vi "Main Page.vi"(8 "error in (no error)":errorcluster, 11 "Node Ptr":T2 format="%.0x") -> (0 "error out":errorcluster)   [LabVIEW 2024, in "Embedded TDMS Logger System Explorer.lvlib"]
doc: "The UI Page giving the user the ability to modify properties on the file level of the custom device, i.e.:\n- Segmentation options\n- Meta Data to be logged on the file level of the TDMS\n- Naming convention of the file\n- Name of the Custom Device\n- Directory to log files into."
uses:
  Embedded TDMS Logger System Explorer.lvlib
  <vilib>/NI VeriStand/Custom Device API/Custom Device Item Ref.ctl
  Shared/SegmentOptions.ctl
  Shared/File Classes/Meta Data.ctl
  <vilib>/NI VeriStand/Custom Device API/Get Item Property (U16).vi
  <vilib>/NI VeriStand/Custom Device API/Get Item Property (Variant).vi
  <vilib>/NI VeriStand/Custom Device API/Set Item Property (Variant).vi
  <vilib>/NI VeriStand/Custom Device API/Set Item Property (U16).vi
  <vilib>/NI VeriStand/Custom Device API/Set Item Property (String).vi
  <vilib>/NI VeriStand/Custom Device API/Set Item Property (Boolean).vi
  <vilib>/NI VeriStand/Custom Device API/Set Item Property (U64).vi
  <vilib>/NI VeriStand/Custom Device API/Custom Device API.lvlib
panel:
  in  "Tab Control":enum32{"File Settings", "Actions", "Meta Data"}(tab)
  out "String 3":string="The data format can be specified in the string, as with the formats specified in: https://www.ni.com/docs/en-US/bundle/labview-api-ref/page/functions/format-date-time-string.html"
  in  "Segment every":dbl=3600.0
  in  "Segment by":T1=enum."Size (MB)"
  in  "Filename Format:":string="mytestfile_%Y-%m-%d-%H-%M-%S.tdms"
  in  "Log Directory":string
  in  "Segment Files":bool=TRUE
  in  "Error Command":string
  in  "Segment Command":string caption="Run Command"
  in  "Start Command":string
  in  "On Error":bool=TRUE
  in  "On Recording":bool=TRUE
  in  "On Segmentation":bool=TRUE
  in  "File Level Meta Data":string[][](table)=[["Software Version"], ["Test Rig Used"], ["UUT"], ["Operator"]]
  in  "Async Timeout (ms)":u16
  out "Version":string
  in  "Specific Header":cluster{"Section Name":string}={"Section Name"="Custom Device Item Settings"}
  in  "General Header":cluster{"Section Name":string}={"Section Name"="General Custom Device Settings"}
  in  "Description":string
  in  "Name":string
  # "Note: For Windows systems as the engine/target we recommend placing your commands in batch files\nand calling with cmd /C start \"\" prepended to detach the process:\n\ncmd /C start \"\" \"C:\\Users\\tq7638\\test.bat\"\n\nNote: You can use [filepath] in the command to substitute in the current/previous filepath recorded.\nFor the error command you can use [error code] to get the error code and [error source] for source."
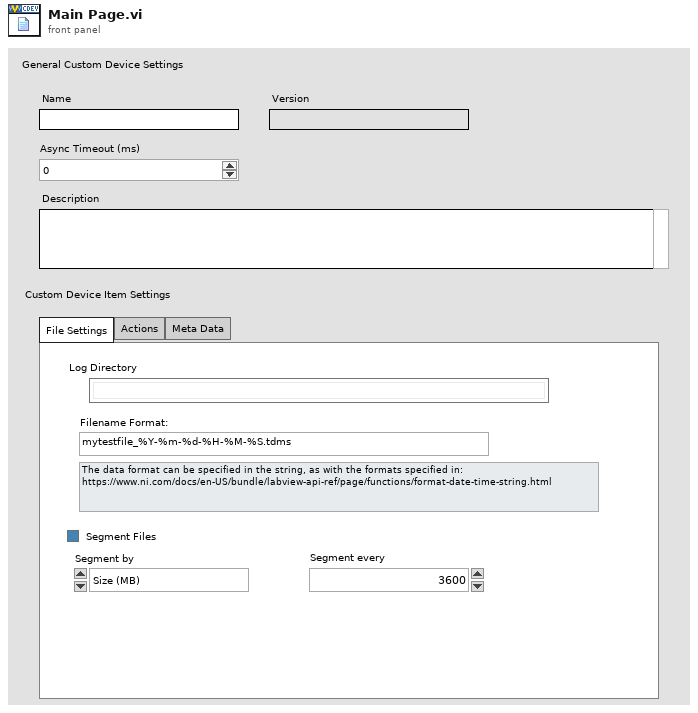
[diagram p1: front panel]
types:
  T1 = typedef "SegmentOptions.ctl" = enum16{"Time (s)", "Size (MB)"}
  T2 = typedef "Custom Device API.lvlib/Custom Device Item Ref.ctl" = u64
  T3 = typedef "Custom Device API.lvlib/Custom Device Item Info.ctl" = cluster{"Name":string, "Is Channel":bool, "GUID":string, "Is Waveform":bool}
  T4 = typedef "Meta Data.ctl" = cluster{"Key":string, "Value":string}
  T5 = typedef "Custom Device API.lvlib/Custom Device Commands.ctl" = enum16{"Default", "Item renamed", "Shutdown", "Dynamic button pressed"}
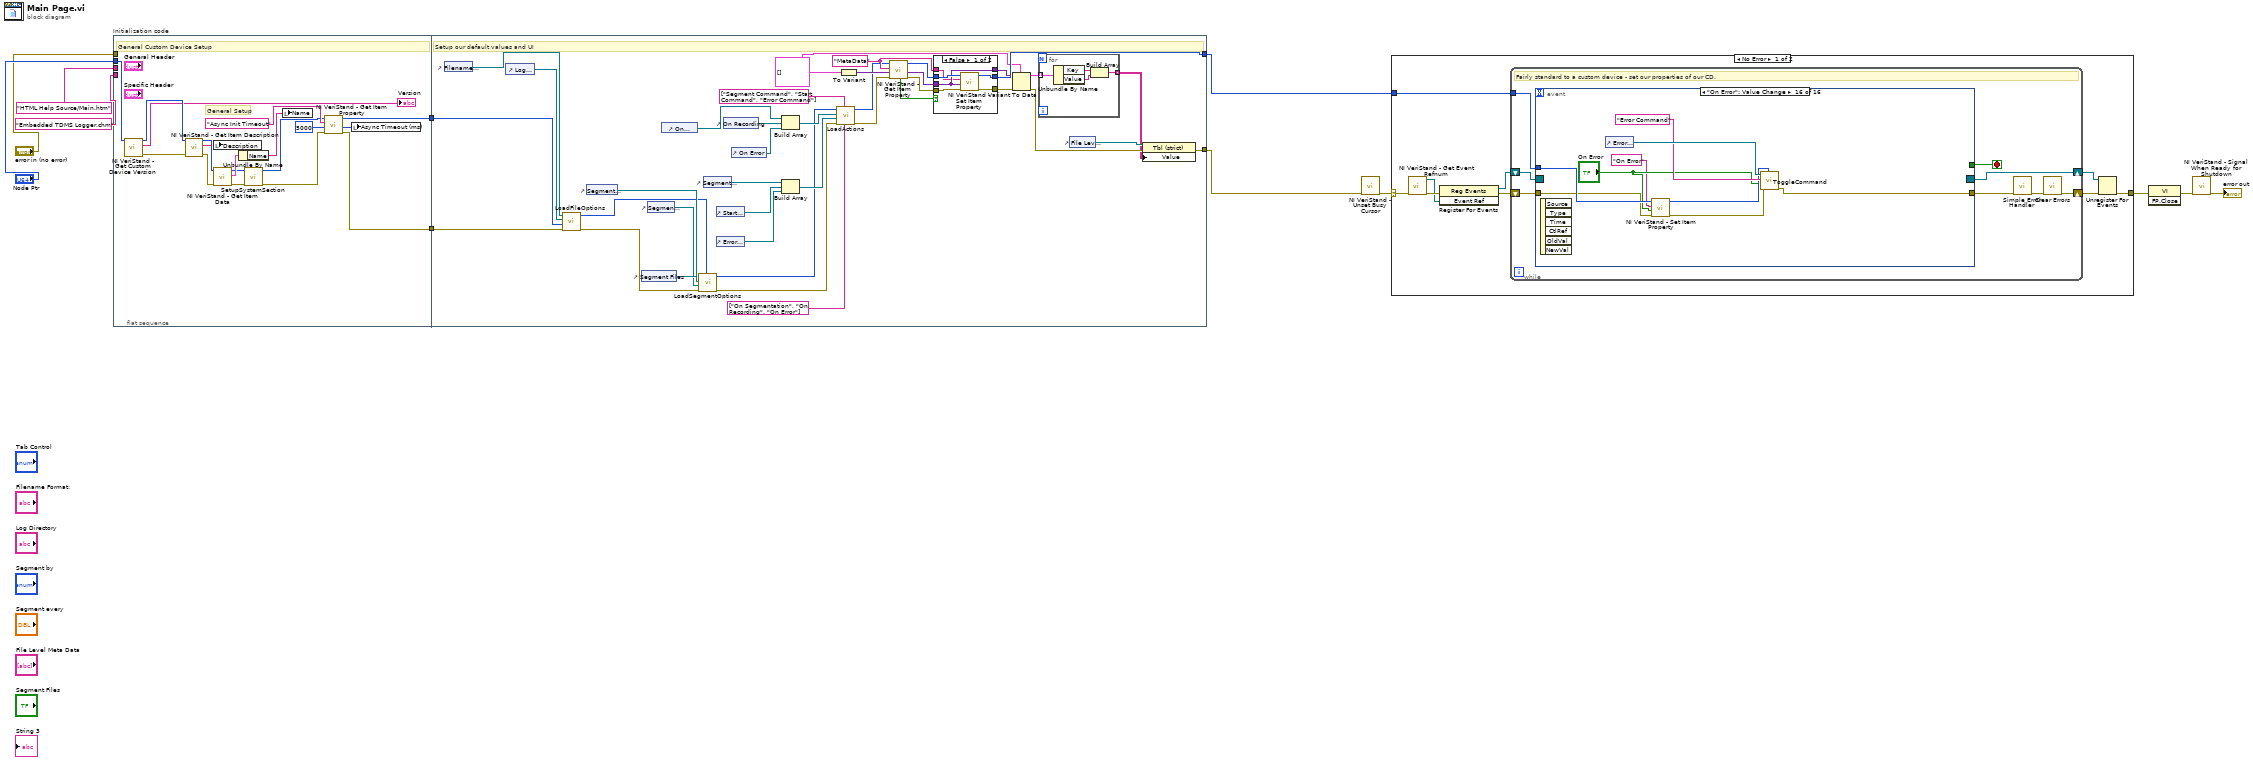
[diagram p0: block diagram]
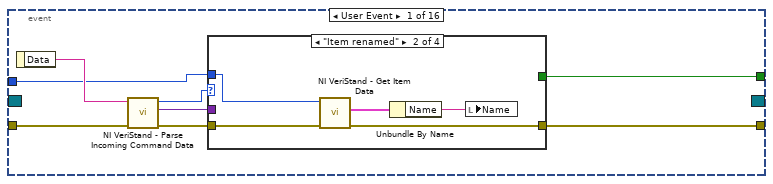
[diagram p2: hidden frame]
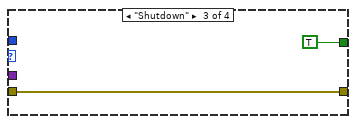
[diagram p4: hidden frame]
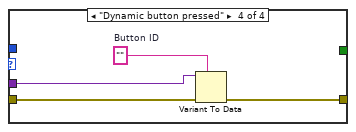
[diagram p5: hidden frame]
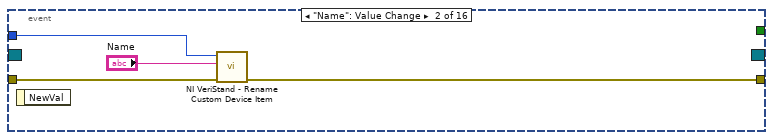
[diagram p6: hidden frame]
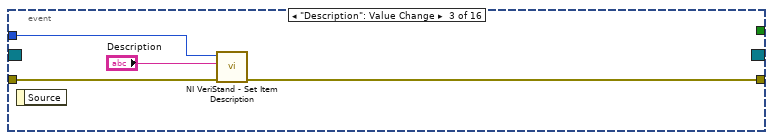
[diagram p7: hidden frame]
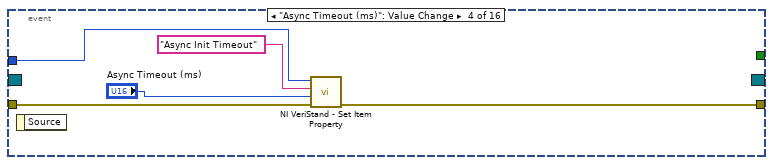
[diagram p8: hidden frame]
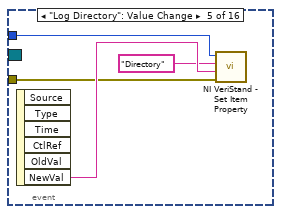
[diagram p9: hidden frame]
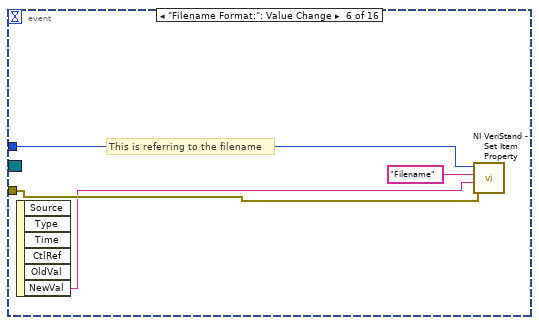
[diagram p10: hidden frame]
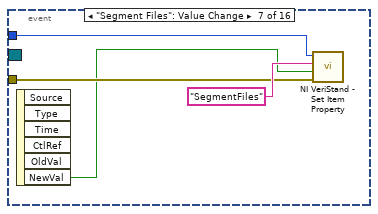
[diagram p11: hidden frame]
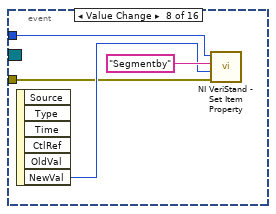
[diagram p12: hidden frame]
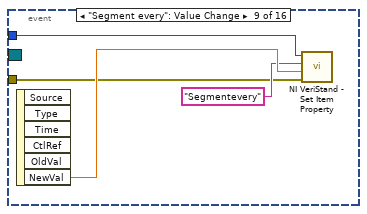
[diagram p13: hidden frame]
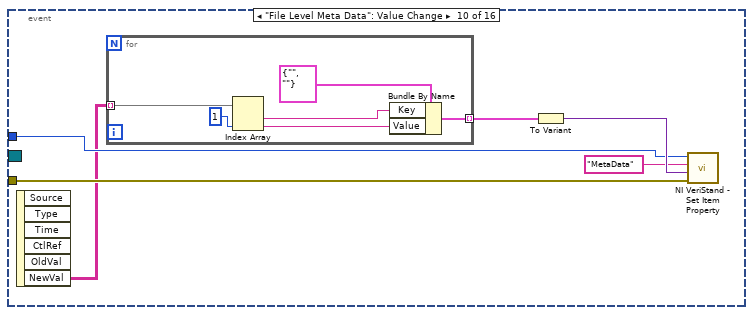
[diagram p14: hidden frame]
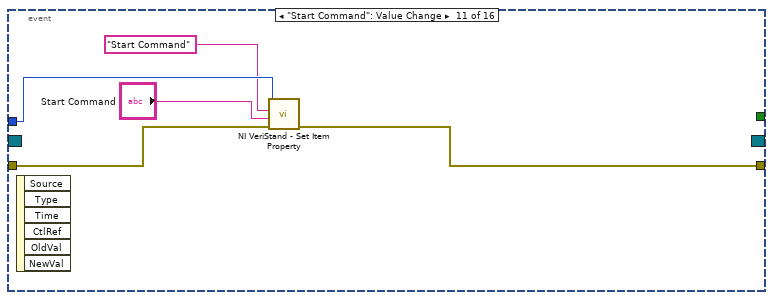
[diagram p15: hidden frame]
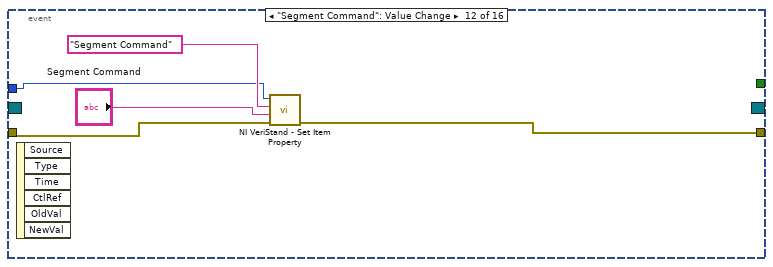
[diagram p16: hidden frame]
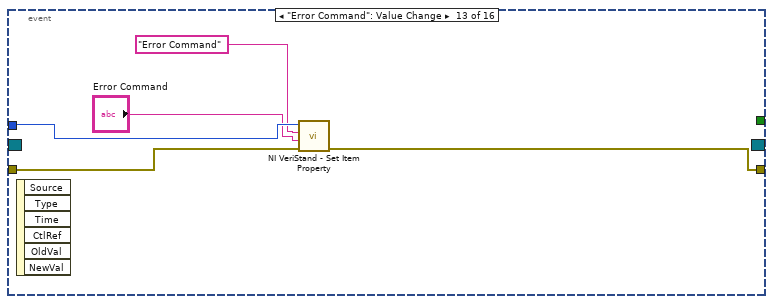
[diagram p17: hidden frame]
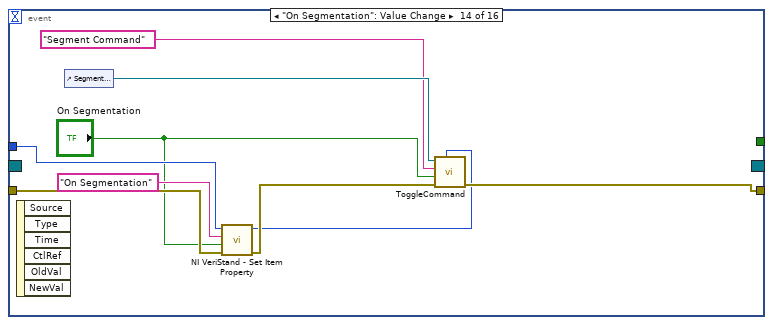
[diagram p18: hidden frame]
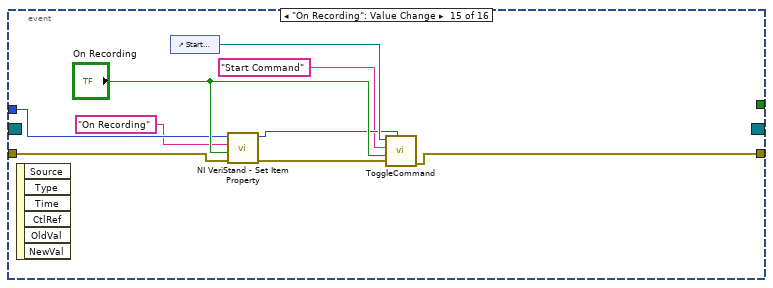
[diagram p19: hidden frame]
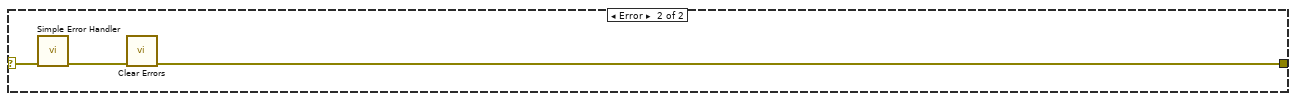
[diagram p20: hidden frame]
diagram:
  n1 = flat-sequence "Initialization code" {
    tunnel: "error in (no error)" -> [_]
    tunnel: "Node Ptr" -> [w27]
    tunnel: "HTML Help Source/Main.htm" ("HTML File") -> [_]
    tunnel: "Embedded TDMS Logger.chm" ("CD_CHM_FileName") -> [_]
    tunnel: [w18] -> w4
    tunnel: [w17] -> w3
    tunnel: w4 -> [w68]
    tunnel: w3 -> [w45]
    tunnel: [w56] -> w2
    tunnel: [w55] -> w1
    frame #0 {
      # "General Setup"
      # "General Custom Device Setup"
      n2 = call <vilib>:"NI VeriStand - Get Custom Device Version.vi"("Device Ref in"=w27) -> ("error out"=w26:errorcluster, "Value"=→"Version":string, "Device Ref out"=w25:T2)  [unwired: 8 in]
      n3 = call <vilib>:"NI VeriStand - Get Item Description.vi"("error in (no error)"=w26, "Item Ref in"=w25) -> ("error out"=w29:errorcluster, "Description"=w22:string, "Item Ref out"=w30:T2)  [unwired: 7 out]
      n4 = local write "Description"(w22) -> ()
      n5 = call <vilib>:"NI VeriStand - Get Item Data.vi"("error in (no error)"=w29, "Item Ref in"=w30) -> ("error out"=w15:errorcluster, "Item Info"=w28:T3, "Item Ref out"=w16:T2)  [unwired: 7 out]
      n6 = Unbundle By Name(w28) -> ("Name"=w23:string)
      n7 = call "SetupSystemSection.vi"("error in (no error)"=w15, "Node Ptr"=w16) -> ("error out"=w14:errorcluster, "Parent Ref Out"=w13:T2)  [unwired: 4 in, 4 out]
      n8 = local write "Name"(w23) -> ()
      n9 = call-poly <vilib>:"NI VeriStand - Get Item Property.vi"("error in (no error)"=w14, "Default Value"=u16 5000, "Property Name"="Async Init Timeout", "Item Ref in"=w13) -> ("error out"=w18:errorcluster, "Value"=w21:u16, "Item Ref out"=w17:T2)  [unwired: 4 in, 1 out]
      n10 = local write "Async Timeout (ms)"(w21) -> ()
    }
    frame #1 {
      w47 = T4[] []
      w54 = "MetaData" ("Property Name")
      # "Setup our default values and UI"
      n11 = control-ref of="Filename Format:"() -> (w67:refnum<vi>)
      n12 = control-ref of="Log Directory"() -> (w46:refnum<vi>)
      n13 = call "LoadFileOptions.vi"("error in (no error)"=w68, "Item Ref in"=w45, "Directory In"=w46, "Filename in"=w67) -> ("error out"=w66:errorcluster, "Item Ref out"=w63:T2)  [unwired: 6 in]
      n14 = control-ref of="Segment every"() -> (w65:refnum<vi>)
      n15 = control-ref of="Segment Files"() -> (w64:refnum<vi>)
      n16 = control-ref of="Segment by"() -> (w62:refnum<vi>)
      n17 = control-ref of="On Segmentation"() -> (w42:refnum<vi>)
      n18 = call "LoadSegmentOptions.vi"("Item Ref in"=w63, "error in (no error)"=w66, "Segment by"=w62, "Segment every"=w65, "Boolean in"=w64) -> ("error out"=w31:errorcluster, "Item Ref out"=w34:T2)  [unwired: 5 in]
      n19 = control-ref of="Segment Command"() -> (w39:refnum<vi>)
      n20 = control-ref of="Start Command"() -> (w40:refnum<vi>)
      n21 = control-ref of="Error Command"() -> (w41:refnum<vi>)
      n22 = control-ref of="On Recording"() -> (w43:refnum<vi>)
      n23 = control-ref of="On Error"() -> (w44:refnum<vi>)
      n24 = Build Array(w42, w43, w44) -> (w38:refnum<vi>[])
      n25 = Build Array(w39, w40, w41) -> (w37:refnum<vi>[])
      n26 = call "LoadActions.vi"("Array 2"=string[] ["On Segmentation", "On Recording", "On Error"], "Array"=string[] ["Segment Command", "Start Command", "Error Command"], "error in (no error)"=w31, "Array 4"=w37, "Array 3"=w38, "Item Ref in"=w34) -> ("error out"=w32:errorcluster, "Item Ref out"=w33:T2)  [unwired: 4 in]
      n27 = To Variant(anything=w47) -> (Variant=w58:variant)
      n28 = call-poly <vilib>:"NI VeriStand - Get Item Property.vi"("error in (no error)"=w32, "Default Value"=w58, "Property Name"=w54, "Item Ref in"=w33) -> ("error out"=w60:errorcluster, "Value"=w59:variant, "Item Ref out"=w57:T2, "Found?"=w61:bool)  [unwired: 4 in]
      n29 = case shown="False" w61 {
        tunnel: [w78 w81] -> w56
        tunnel: w57 -> [w77 w81]
        tunnel: [w76 w80] -> w52
        tunnel: w60 -> [w75 w80]
        tunnel: w59 -> [w74 w79]
        tunnel: [w74 w79] -> w50
        tunnel: w54 -> [w73 _]
        frame False {
          n30 = call-poly <vilib>:"NI VeriStand - Set Item Property.vi"("error in (no error)"=w75, "Value"=w74, "Property Name"=w73, "Item Ref in"=w77) -> ("error out"=w76:errorcluster, "Item Ref out"=w78:T2)  [unwired: 5 in, 1 out]
        }
        frame True {
        }
      }
      n31 = Variant To Data(error in=w52, type=w47, Variant=w50) -> (data=w48:T4[], error out=w51:errorcluster)
      n32 = for {
        tunnel: [w70] -> w49 mode=indexing
        tunnel: w48 -> [w69] mode=indexing
        n33 = Unbundle By Name(w69) -> ("Key"=w72:string, "Value"=w71:string)
        n34 = Build Array(w72, w71) -> (w70:string[])
      }
      n35 = control-ref of="File Level Meta Data"() -> (w53:refnum<vi>)
      n36 = property class="Tbl (strict)"(reference=w53, error in=w51, "Value"=w49) -> (error out=w55:errorcluster)  [unwired: 1 out]
    }
  }
  n37 = call <vilib>:"NI VeriStand - Unset Busy Cursor.vi"("error in (no error)"=w1) -> ("error out"=w8:errorcluster)  [unwired: 10 out]
  n38 = case shown="No Error" w8 {
    selector: w8 -> [w83 w208]
    tunnel: [w87 w206] -> w12
    tunnel: w2 -> [w82 _]
    frame No Error {
      n39 = call <vilib>:"NI VeriStand - Get Event Refnum.vi"("error in (no error)"=w83) -> ("error out"=w90:errorcluster, "Event Ref"=w86:refnum<user-event>)  [unwired: 9 out]
      n40 = register-events(error in=w90, w86) -> (reference out=w84:refnum<event-registration>, error out=w85:errorcluster)  [unwired: 1 in]
      n41 = while {
        shift-right: [w92] -> w88
        shift-left: w85 -> [w97]
        shift-right: [w98] -> w89
        shift-left: w84 -> [w96]
        tunnel: w82 -> [w91]
        stop <- w95 stop-if-true
        # "Fairly standard to a custom device - set our properties of our CD."
        n42 = event shown="[15] \"On Error\": Value Change" {
          selector: w96 -> [_ _ _ _ _ _ _ _ _ _ _ _ _ _ _ _]
          dyn-events: [_ _ _ _ _ _ _ _ _ _ _ _ _ _ _ _] -> w98
          timeout: _ -> [_ _ _ _ _ _ _ _ _ _ _ _ _ _ _ _]
          tunnel: w97 -> [w106 w122 w126 w131 w133 w138 w142 w144 w148 w154 w168 w173 w175 w184 w190 w199]
          tunnel: [w102 _ _ _ _ _ _ _ _ _ _ _ _ _ _ _] -> w95
          tunnel: [w101 w121 w125 w129 _ _ _ _ _ _ w165 w169 w174 w186 w195 w205] -> w94
          tunnel: w91 -> [w99 w119 w123 w127 w132 w136 w141 w145 w150 w155 w166 w170 w178 w182 w191 w202]
          event User Event {
            n43 = event-data() -> ("Data"=w105:string)  [unwired: 1 out]
            n44 = call <vilib>:"NI VeriStand - Parse Incoming Command Data.vi"("error in (no error)"=w106, "Incoming data"=w105) -> ("error out"=w104:errorcluster, "Outgoing data"=w100:variant, "Action"=w103:T5)  [unwired: 7 out]
            n45 = case shown="\"Item renamed\"" w103 {
              tunnel: w104 -> [w107 w112 w113 w118]
              tunnel: [_ _ TRUE _] -> w102
              tunnel: [w107 w110 w113 w115] -> w101
              tunnel: w100 -> [_ _ _ w117]
              tunnel: w99 -> [_ w108 _ _]
              frame "Default", Default {
              }
              frame "Item renamed" {
                n46 = call <vilib>:"NI VeriStand - Get Item Data.vi"("error in (no error)"=w112, "Item Ref in"=w108) -> ("error out"=w110:errorcluster, "Item Info"=w111:T3)  [unwired: 8 out]
                n47 = Unbundle By Name(w111) -> ("Name"=w109:string)
                n48 = local write "Name"(w109) -> ()
              }
              frame "Shutdown" {
              }
              frame "Dynamic button pressed" {
                w116 = ""  # Button ID
                n49 = Variant To Data(error in=w118, type=w116, Variant=w117) -> (error out=w115:errorcluster)  [unwired: 1 out]
              }
            }
          }
          event "Name": Value Change {
            n50 = event-data() -> ()  [unwired: 2 out]
            n51 = call <vilib>:"NI VeriStand - Rename Custom Device Item.vi"("error in (no error)"=w122, "New Name"="Name", "Item Ref in"=w119) -> ("error out"=w121:errorcluster)  [unwired: 1 in, 7 out]
          }
          event "Description": Value Change {
            n52 = event-data() -> ()  [unwired: 2 out]
            n53 = call <vilib>:"NI VeriStand - Set Item Description.vi"("error in (no error)"=w126, "Description"="Description", "Item Ref in"=w123) -> ("error out"=w125:errorcluster)  [unwired: 8 out]
          }
          event "Async Timeout (ms)": Value Change {
            n54 = event-data() -> ()  [unwired: 2 out]
            n55 = call-poly <vilib>:"NI VeriStand - Set Item Property.vi"("error in (no error)"=w131, "Value"="Async Timeout (ms)", "Property Name"="Async Init Timeout", "Item Ref in"=w127) -> ("error out"=w129:errorcluster)  [unwired: 5 in, 2 out]
          }
          event "Log Directory": Value Change {
            n56 = event-data() -> ("NewVal"=w135:string)  [unwired: 6 out]
            n57 = call-poly <vilib>:"NI VeriStand - Set Item Property.vi"("error in (no error)"=w133, "Value"=w135, "Property Name"="Directory", "Item Ref in"=w132) -> ()  [unwired: 5 in, 3 out]
          }
          event "Filename Format:": Value Change {
            # "This is referring to the filename"
            n58 = event-data() -> ("NewVal"=w137:string)  [unwired: 6 out]
            n59 = call-poly <vilib>:"NI VeriStand - Set Item Property.vi"("error in (no error)"=w138, "Value"=w137, "Property Name"="Filename", "Item Ref in"=w136) -> ()  [unwired: 5 in, 3 out]
          }
          event "Segment Files": Value Change {
            n60 = event-data() -> ("NewVal"=w140:bool)  [unwired: 6 out]
            n61 = call-poly <vilib>:"NI VeriStand - Set Item Property.vi"("error in (no error)"=w142, "Value"=w140, "Property Name"="SegmentFiles", "Item Ref in"=w141) -> ()  [unwired: 5 in, 3 out]
          }
          event Value Change {
            n62 = event-data() -> ("NewVal"=w146:T1)  [unwired: 6 out]
            n63 = call-poly <vilib>:"NI VeriStand - Set Item Property.vi"("error in (no error)"=w144, "Value"=w146, "Property Name"="Segmentby", "Item Ref in"=w145) -> ()  [unwired: 5 in, 3 out]
          }
          event "Segment every": Value Change {
            n64 = event-data() -> ("NewVal"=w151:dbl)  [unwired: 6 out]
            n65 = call-poly <vilib>:"NI VeriStand - Set Item Property.vi"("error in (no error)"=w148, "Value"=w151, "Property Name"="Segmentevery", "Item Ref in"=w150) -> ()  [unwired: 5 in, 3 out]
          }
          event "File Level Meta Data": Value Change {
            n66 = event-data() -> ("NewVal"=w152:string[][])  [unwired: 6 out]
            n67 = for {
              tunnel: [w163] -> w153 mode=indexing
              tunnel: w152 -> [w159] mode=indexing
              n68 = Index Array(array=w159, index #2=1 ("index")) -> (element #1=w160:string, element #2=w161:string)  [unwired: 1 in]
              n69 = Bundle By Name(cluster=T4 {"Key"="", "Value"=""} ("Meta Data"), "Key"=w160, "Value"=w161) -> (w163:T4)
            }
            n70 = To Variant(anything=w153) -> (Variant=w157:variant)
            n71 = call-poly <vilib>:"NI VeriStand - Set Item Property.vi"("error in (no error)"=w154, "Value"=w157, "Property Name"="MetaData", "Item Ref in"=w155) -> ()  [unwired: 5 in, 3 out]
          }
          event "Start Command": Value Change {
            n72 = event-data() -> ()  [unwired: 7 out]
            n73 = call-poly <vilib>:"NI VeriStand - Set Item Property.vi"("error in (no error)"=w168, "Value"="Start Command", "Property Name"="Start Command", "Item Ref in"=w166) -> ("error out"=w165:errorcluster)  [unwired: 5 in, 2 out]
          }
          event "Segment Command": Value Change {
            n74 = event-data() -> ()  [unwired: 7 out]
            n75 = call-poly <vilib>:"NI VeriStand - Set Item Property.vi"("error in (no error)"=w173, "Value"="Segment Command", "Property Name"="Segment Command", "Item Ref in"=w170) -> ("error out"=w169:errorcluster)  [unwired: 5 in, 2 out]
          }
          event "Error Command": Value Change {
            n76 = event-data() -> ()  [unwired: 7 out]
            n77 = call-poly <vilib>:"NI VeriStand - Set Item Property.vi"("error in (no error)"=w175, "Value"="Error Command", "Property Name"="Error Command", "Item Ref in"=w178) -> ("error out"=w174:errorcluster)  [unwired: 5 in, 2 out]
          }
          event "On Segmentation": Value Change {
            n78 = event-data() -> ()  [unwired: 7 out]
            n79 = control-ref of="Segment Command"() -> (w187:refnum<vi>)
            n80 = call-poly <vilib>:"NI VeriStand - Set Item Property.vi"("error in (no error)"=w184, "Value"="On Segmentation", "Property Name"="On Segmentation", "Item Ref in"=w182) -> ("error out"=w183:errorcluster, "Item Ref out"=w181:T2)  [unwired: 5 in, 1 out]
            n81 = call "ToggleCommand.vi"("Item Ref in"=w181, "error in (no error)"=w183, "On Segmentation"="On Segmentation", "Property Name"="Segment Command", "String in"=w187) -> ("error out"=w186:errorcluster)  [unwired: 6 in]
          }
          event "On Recording": Value Change {
            n82 = event-data() -> ()  [unwired: 7 out]
            n83 = control-ref of="Start Command"() -> (w193:refnum<vi>)
            n84 = call-poly <vilib>:"NI VeriStand - Set Item Property.vi"("error in (no error)"=w190, "Value"="On Recording", "Property Name"="On Recording", "Item Ref in"=w191) -> ("error out"=w196:errorcluster, "Item Ref out"=w192:T2)  [unwired: 5 in, 1 out]
            n85 = call "ToggleCommand.vi"("Item Ref in"=w192, "error in (no error)"=w196, "On Segmentation"="On Recording", "Property Name"="Start Command", "String in"=w193) -> ("error out"=w195:errorcluster)  [unwired: 6 in]
          }
          event "On Error": Value Change {
            n86 = event-data() -> ()  [unwired: 7 out]
            n87 = control-ref of="Error Command"() -> (w204:refnum<vi>)
            n88 = call-poly <vilib>:"NI VeriStand - Set Item Property.vi"("error in (no error)"=w199, "Value"="On Error", "Property Name"="On Error", "Item Ref in"=w202) -> ("error out"=w200:errorcluster, "Item Ref out"=w201:T2)  [unwired: 5 in, 1 out]
            n89 = call "ToggleCommand.vi"("Item Ref in"=w201, "error in (no error)"=w200, "On Segmentation"="On Error", "Property Name"="Error Command", "String in"=w204) -> ("error out"=w205:errorcluster)  [unwired: 6 in]
          }
        }
        n90 = call <vilib>:"Simple Error Handler.vi"("error in (no error)"=w94) -> ("error out"=w93:errorcluster)  [unwired: 1 in, 7 out]
        n91 = call <vilib>:"Clear Errors.vi"("error in (no error)"=w93) -> ("error out"=w92:errorcluster)  [unwired: 1 in, 5 out]
      }
      n92 = Unregister For Events(event registration refnum=w89, error in=w88) -> (error out=w87:errorcluster)
    }
    frame Error {
      n93 = call <vilib>:"Simple Error Handler.vi"("error in (no error)"=w208) -> ("error out"=w207:errorcluster)  [unwired: 1 in, 7 out]
      n94 = call <vilib>:"Clear Errors.vi"("error in (no error)"=w207) -> ("error out"=w206:errorcluster)  [unwired: 1 in, 5 out]
    }
  }
  n95 = invoke class="VI" method="FP.Close"(error in=w12) -> (error out=w11:errorcluster)  [unwired: 2 in, 2 out]
  n96 = call <vilib>:"NI VeriStand - Signal When Ready for Shutdown.vi"("error in (no error)"=w11) -> ("error out"=→"error out":errorcluster)  [unwired: 10 out]
